vi "CreateFilePath.vi"(10 "Suffix":i32, 11 "base path":path=path "C:/Users/Bruce Wayne/Desktop/SourceCode_20171218/thresholds.csv") -> (3 "appended path":path)   [LabVIEW 2018]
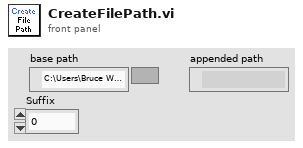
[diagram p1: front panel]
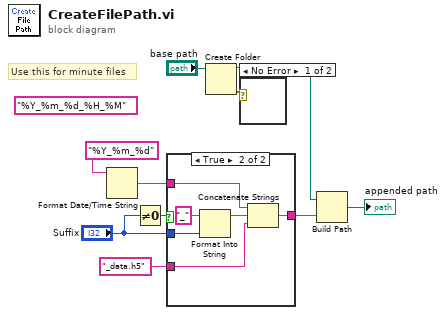
[diagram p0: block diagram]
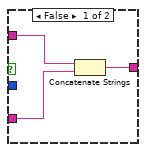
[diagram p2: hidden frame]
diagram:
  (unwired) "%Y_%m_%d_%H_%M" ("time format string (%c)")
  # "Use this for minute files"
  n1 = Format Date/Time String(time format string (%c)="%Y_%m_%d") -> (date/time string=w5:string)  [unwired: 2 in]
  n2 = Not Equal To 0?(x="Suffix") -> (x != 0?=w2:bool)
  n3 = case shown="True" w2 {
    tunnel: "_data.h5" ("string") -> [w12 w19]
    tunnel: w5 -> [w13 w18]
    tunnel: [w11 w17] -> w4
    tunnel: "Suffix" -> [_ w16]
    frame False {
      n4 = Concatenate Strings(w13, w12) -> (w11:string)
    }
    frame True {
      n5 = Format Into String(initial string="_" ("string"), w16) -> (resulting string=w14:string)  [unwired: 2 in, 1 out]
      n6 = Concatenate Strings(w18, w14, w19) -> (w17:string)
    }
  }
  n7 = Create Folder(path (use dialog)="base path") -> (created path=w10:path, error out=w7:errorcluster)  [unwired: 2 in, 1 out]
  n8 = case shown="No Error" w7 {
    frame No Error {
    }
    frame Error {
    }
  }
  n9 = Build Path(base path=w10, name or relative path=w4) -> (appended path=→"appended path":path)
